vi "Update Test Name.vi"(8 "error in":errorcluster, 10 "Test_Name":string, 11 "Report Generator in":refnum<class "Report Generator.lvclass">) -> (0 "error out":errorcluster, 3 "Report Generator out":refnum<class "Report Generator.lvclass">)   [LabVIEW 2019, in "Report Generator.lvlib" / "Report Generator.lvclass"]
uses:
  Library/Report Generator.lvclass
  C:/Users/Public/Documents/Development/builds/Engine/Engine.lvlibp/Project/Engine.lvclass
  builds/Engine/Actor Framework.lvlibp/1abvi3w/vi.lib/ActorFramework/Message Enqueuer/Message Priority.ctl
  Library/Report Generator.lvclass/Report Generator.ctl
  builds/Engine/Engine.lvlibp/Accessors/Read Report Queue.vi
  builds/Engine/Engine.lvlibp/Accessors/Read Self Q.vi
  builds/Engine/Actor Framework.lvlibp/1abvi3w/vi.lib/ActorFramework/Message Enqueuer/Enqueue.vi
  builds/Tools/QDMH.lvlibp/Private/Enqueue Unbundled Element.vi
  builds/Tools/QDMH.lvlibp/QDMH.lvclass
  builds/Engine/Actor Framework.lvlibp/1abvi3w/vi.lib/ActorFramework/Message Enqueuer/Message Enqueuer.lvclass
  Report Generator Messages/Prepare Test Naming Msg/Prepare Test Naming Msg.lvclass
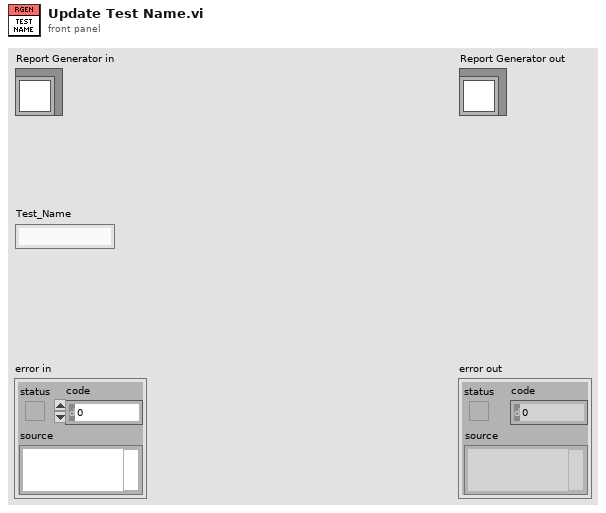
[diagram p1: front panel]
types:
  T1 = typedef "Actor Framework.lvlibp/Message Enqueuer.lvclass/Message Priority.ctl" = enum16{"Low", "Normal", "High"}
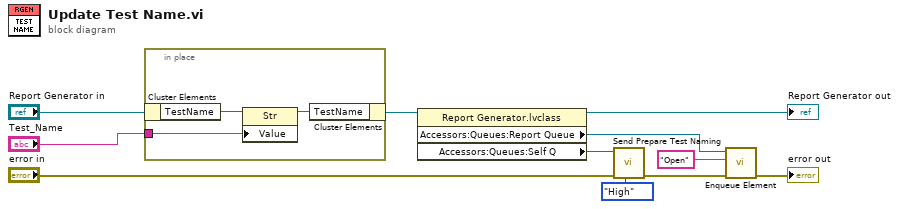
[diagram p0: block diagram]
diagram:
  n1 = in-place {
    in-place-border: "Test_Name" -> [w13]
    n2 = in-place-cluster #1("Report Generator in") -> ("TestName"=w14:refnum<vi>)
    n3 = property class="Str"(reference=w14, "Value"=w13) -> (reference out=w12:refnum<vi>)  [unwired: 1 in, 1 out]
    n4 = in-place-cluster #1("TestName"=w12) -> (w9:refnum<class "Report Generator.lvclass">)
  }
  n5 = property class="Report Generator.lvclass"(reference=w9) -> (reference out=→"Report Generator out":refnum<class "Report Generator.lvclass">, "Accessors:Queues:Report Queue"=w5:refnum<class "QDMH.lvclass">, "Accessors:Queues:Self Q"=w7:refnum<class "Message Enqueuer.lvclass">)  [unwired: 1 in, 1 out]
  n6 = call "Send Prepare Test Naming.vi"("Message Priority (Normal)"=Message_Priority."High", "error in (no error)"="error in", "Message Enqueuer"=w7) -> ("error out"=w3:errorcluster)  [unwired: 7 in, 1 out]
  n7 = call-poly "Enqueue Element.vi"("error in"=w3, "State"="Open", "QDMH in"=w5) -> ("error out"=→"error out":errorcluster)  [unwired: 7 in, 1 out]
